vi "Sim_Control.vi"() -> ()   [LabVIEW 2009]
panel:
  in  "Compass Error (deg)":dbl=0.3
  out "Heading Chart":dbl(graph)
  out "Compass Heading":dbl=1.0
  in  "Compass Update Rate":dbl=8.0
  in  "Iterations?":bool
  in  "Iterations":i32=300
  in  "Initial Paremeters":T1={"X"=0.0, "Vx"=0.0, "Ax"=0.0, "Y"=0.0, "Vy"=0.0, "Ay"=0.0, "Theta"=-90.0, "Omega"=0.0, "Alpha"=0.0}
  in  "Enable Step?":bool
  in  "step":bool
  in  "Motor Voltages":cluster{"Left Voltage":dbl, "Right Voltage":dbl}={"Left Voltage"=5.0, "Right Voltage"=5.0}
  out "XY Graph":T2(graph)
  out "Output Telemetry":T1
  in  "stop":bool
  out "Waveform Chart":T1(graph)
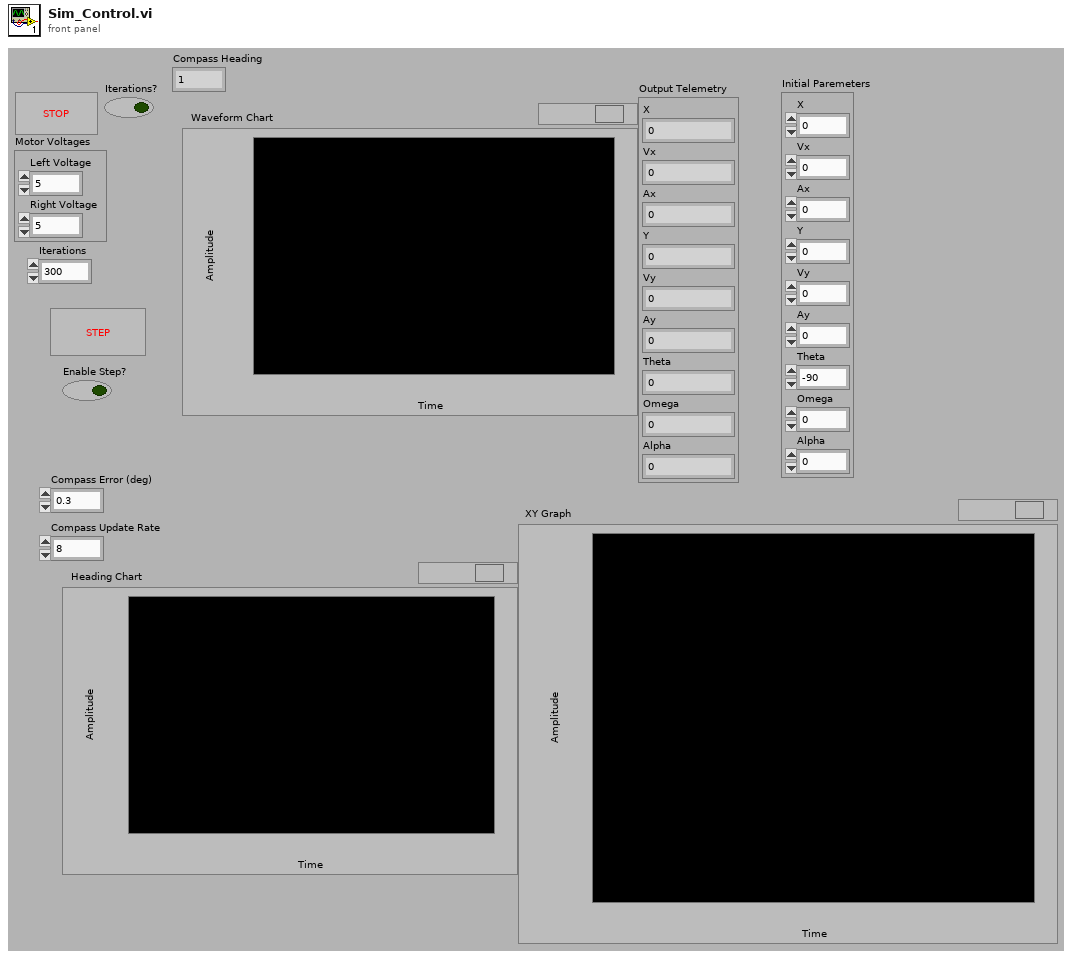
[diagram p1: front panel]
types:
  T1 = cluster{"X":dbl, "Vx":dbl, "Ax":dbl, "Y":dbl, "Vy":dbl, "Ay":dbl, "Theta":dbl, "Omega":dbl, "Alpha":dbl}
  T2 = cluster{"initialized array":dbl[], "initialized array":dbl[]}[]
  T3 = cluster{"X":dbl, "Vx":dbl, "Ax":dbl, "Y":dbl, "Vy":dbl, "Ay":dbl, "Theta":dbl, "Omega":dbl, "Alpha":dbl}[]
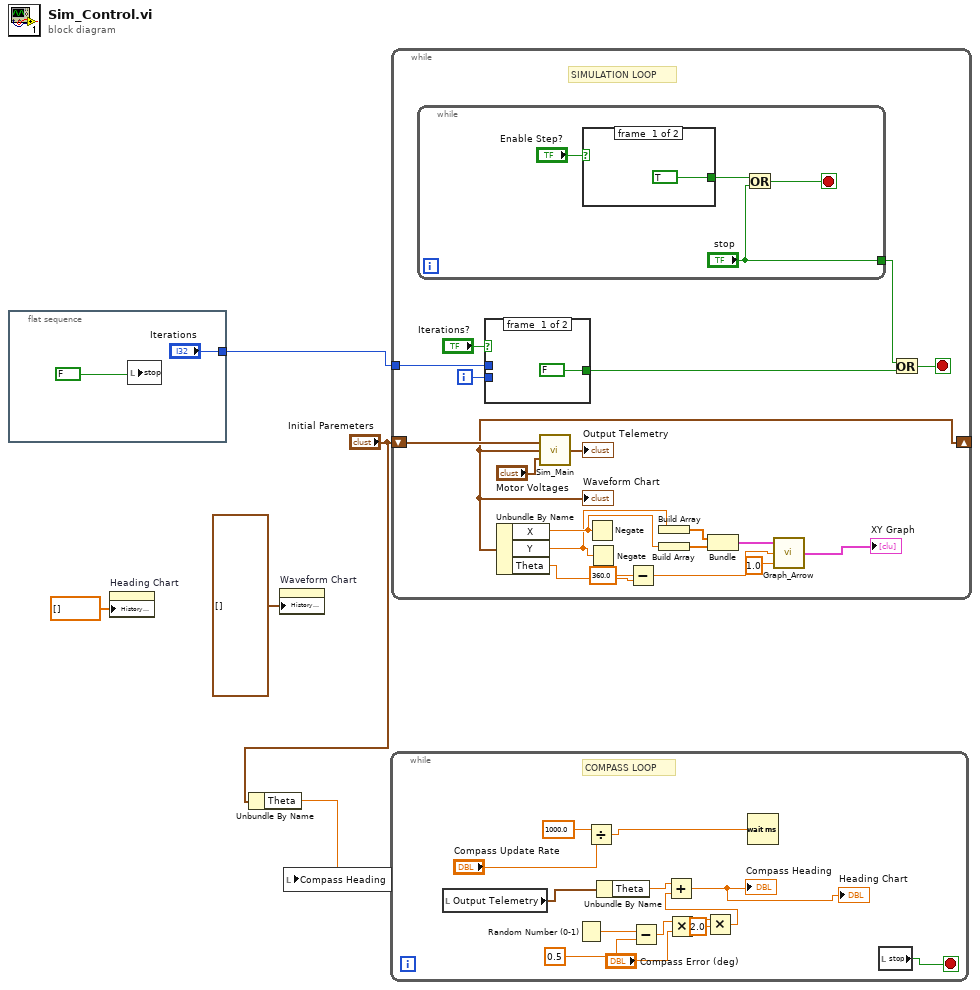
[diagram p0: block diagram]
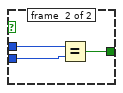
[diagram p2: hidden frame]
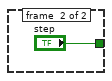
[diagram p3: hidden frame]
diagram:
  n1 = flat-sequence {
    tunnel: ["Iterations"] -> w4
    frame #0 {
      n2 = local write "stop"(FALSE) -> ()
    }
  }
  n3 = property on="Heading Chart" class="WFChart (strict)"("History Data"=dbl[] []) -> ()  [unwired: 2 in, 2 out]
  n4 = Unbundle By Name("Initial Paremeters") -> ("Theta"=w2:dbl)
  n5 = property on="Waveform Chart" class="WFChart (strict)"("History Data"=T3 []) -> ()  [unwired: 2 in, 2 out]
  n6 = local write "Compass Heading"(w2) -> ()
  n7 = while {
    stop <- w18 stop-if-true
    # "COMPASS LOOP"
    n8 = local read "Output Telemetry"() -> (w17:T1)
    n9 = Random Number (0-1)() -> (number: 0 to 1=w16:dbl)
    n10 = Divide(x=1000.0, y="Compass Update Rate") -> (x/y=w19:dbl)
    n11 = Unbundle By Name(w17) -> ("Theta"=w12:dbl)
    n12 = Subtract(x=w16, y=0.5) -> (x-y=w14:dbl)
    n13 = Multiply(x=w14, y="Compass Error (deg)") -> (x*y=w10:dbl)
    n14 = Multiply(x=w10, y=2.0) -> (x*y=w9:dbl)
    n15 = Add(x=w12, y=w9) -> (x+y=→"Compass Heading" →"Heading Chart":dbl)
    n16 = Wait (ms)(milliseconds to wait=w19) -> ()  [unwired: 1 out]
    n17 = local read "stop"() -> (w18:bool)
  }
  n18 = while {
    shift-right: [w37] -> _
    shift-left: "Initial Paremeters" -> [w40]
    tunnel: w4 -> [w29]
    i -> [w31]
    stop <- w32 stop-if-true
    # "SIMULATION LOOP"
    n19 = while {
      tunnel: ["stop"] -> w33
      stop <- w47 stop-if-true
      n20 = case shown="True" "Enable Step?" {
        tunnel: [TRUE ("step") "step"] -> w48
        frame #0 {
        }
        frame #1 {
        }
      }
      n21 = Or(x=w48, y="stop") -> (x .or. y?=w47:bool)
    }
    n22 = case shown="False" "Iterations?" {
      tunnel: w31 -> [_ w44]
      tunnel: [FALSE w43] -> w30
      tunnel: w29 -> [_ w42]
      frame #0 {
      }
      frame #1 {
        n23 = Equal?(x=w42, y=w44) -> (x = y?=w43:bool)
      }
    }
    n24 = call "Sim_Main.vi"("Motor Voltages"="Motor Voltages", "Input Telemetry"=w40) -> ("Output Telemetry"=w37:T1)
    "Waveform Chart" <- w37
    "Output Telemetry" <- w37
    n25 = Unbundle By Name(w37) -> ("X"=w26:dbl, "Y"=w25:dbl, "Theta"=w24:dbl)
    n26 = Negate(x=w26) -> ()  [unwired: 1 out]
    n27 = Negate(x=w25) -> ()  [unwired: 1 out]
    n28 = Subtract(x=360.0, y=w24) -> (x-y=w22:dbl)
    n29 = Build Array(w25) -> (w35:dbl[])
    n30 = Build Array(w26) -> (w34:dbl[])
    n31 = Bundle(w35, w34) -> (w27:cluster{dbl[], dbl[]})  [unwired: 1 in]
    n32 = call "Graph_Arrow.vi"("magnitude"=1.0, "Heading"=w22, "plot data"=w27) -> ("XY Graph"=→"XY Graph":T2)
    n33 = Or(x=w33, y=w30) -> (x .or. y?=w32:bool)
  }
